vi "Get CAN Task Execution State.vi"(8 "error in":errorcluster, 11 "CANopen Master in":refnum<class "CANopen Master.lvclass">) -> (0 "error out":errorcluster, 2 "Execution:State":T1(ring), 3 "CANopen Master out":refnum<class "CANopen Master.lvclass">)   [LabVIEW 2024, in "CANopen Master.lvlib" / "CANopen Master.lvclass"]
uses:
  CANopen Master.lvclass
  CANopen Master.lvclass/CANopen Master.ctl
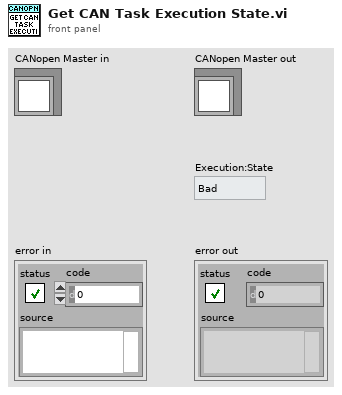
[diagram p1: front panel]
types:
  T1 = enum32{"Bad", "Idle", "Run top level", "Running"}
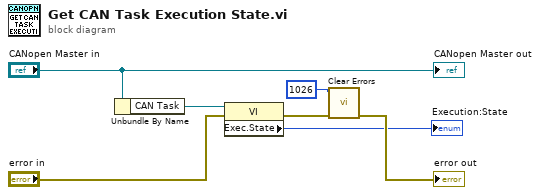
[diagram p0: block diagram]
diagram:
  n1 = Unbundle By Name("CANopen Master in") -> ("CAN Task"=w6:refnum<vi>)
  n2 = property class="VI"(reference=w6, error in="error in") -> (error out=w4:errorcluster, "Exec.State"=→"Execution:State":T1)  [unwired: 1 out]
  n3 = call <vilib>:"Clear Errors.vi"("error in (no error)"=w4, "specific error code to clear (0: all)"=1026) -> ("error out"=→"error out":errorcluster)  [unwired: 4 in, 1 out]
  "CANopen Master out" <- "CANopen Master in"
